vi "ConvertPairSensorReference.vi"(9 "channels":T2[](array[typedef]), 10 "node properties":T1[](array[typedef]), 11 "chan properties in":T1[](array[typedef])) -> (3 "chan properties out":T1[](array[typedef]))   [LabVIEW 2017, in "ServerComm.lvlib"]
uses:
  <vilib>/addons/InsightCM/Devices/Shared/Common/ServerComm/ServerComm.lvlib
  <vilib>/addons/InsightCM/MessageBus/Base/controls/R2_Channel.ctl
  <vilib>/addons/InsightCM/MessageBus/Base/controls/KeyValuePair.ctl
  <vilib>/addons/InsightCM/MessageBus/Base/controls/Metric.ctl
  <vilib>/addons/InsightCM/Utilities/PropertyHelpers/PropertyHelpers.lvlib
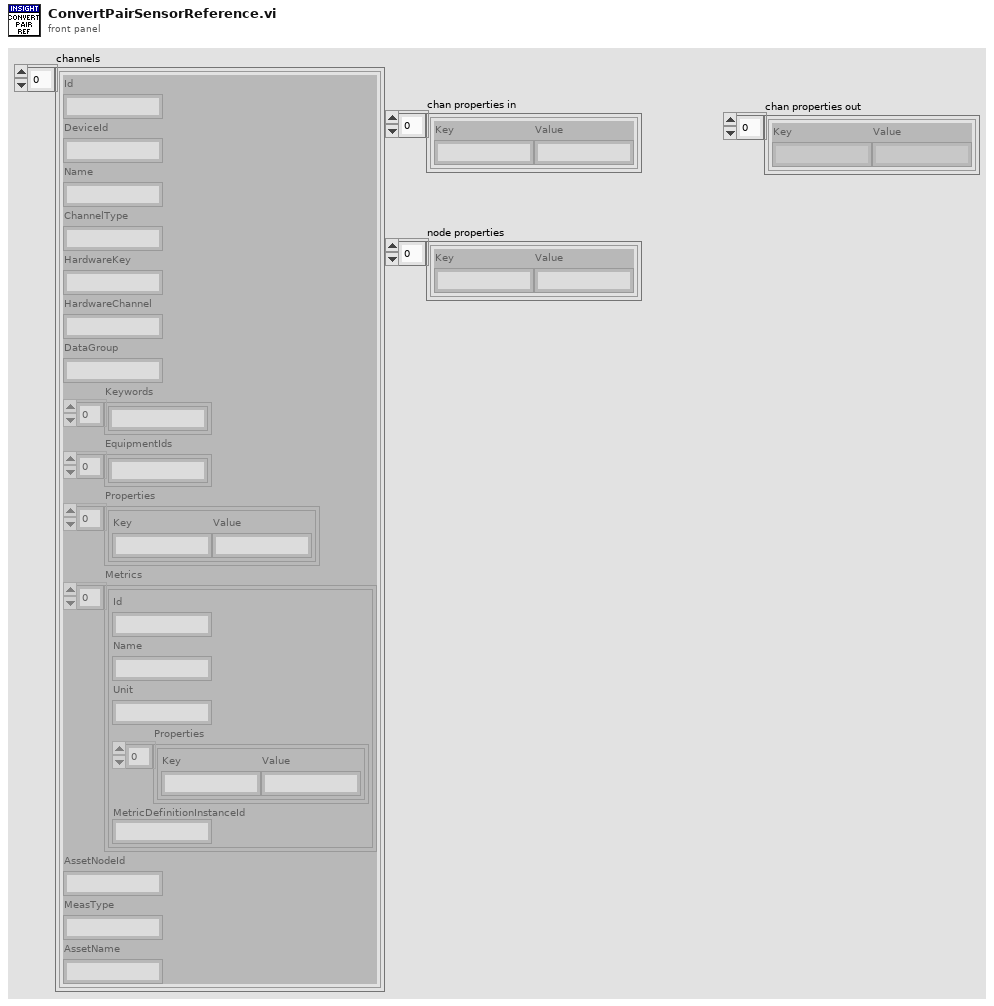
[diagram p1: front panel]
types:
  T1 = typedef "KeyValuePair.ctl" = cluster{"Key":string, "Value":string}
  T2 = typedef "R2_Channel.ctl" = cluster{"Id":string, "DeviceId":string, "Name":string, "ChannelType":string, "HardwareKey":string, "HardwareChannel":string, "DataGroup":string, "Keywords":string[], "EquipmentIds":string[], "Properties":T1[], "Metrics":T3[], "AssetNodeId":string, "MeasType":string, "AssetName":string}
  T3 = typedef "Metric.ctl" = cluster{"Id":string, "Name":string, "Unit":string, "Properties":T1[], "MetricDefinitionInstanceId":string}
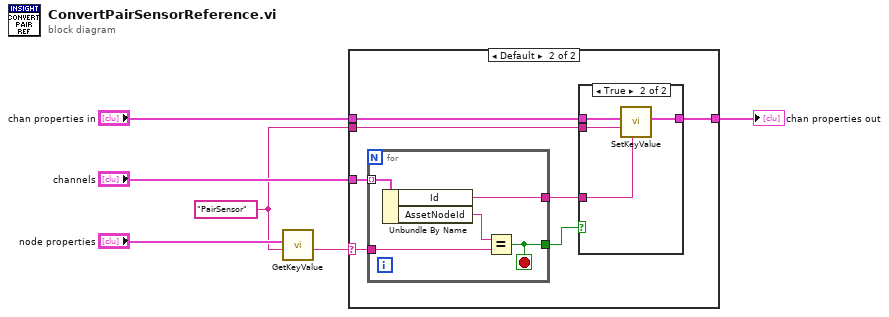
[diagram p0: block diagram]
diagram:
  w2 = "PairSensor" ("key")
  n1 = call <vilib>:"GetKeyValue.vi"("key"=w2, "key value pairs"="node properties") -> ("value"=w4:string)  [unwired: 7 in, 2 out]
  n2 = case shown="Default" w4 {
    selector: w4 -> [_ w13]
    tunnel: "channels" -> [_ w14]
    tunnel: "chan properties in" -> [w7 w11]
    tunnel: w2 -> [_ w10]
    tunnel: [w7 w8] -> w1
    frame "" {
    }
    frame Default {
      n3 = for {
        tunnel: w14 -> [w24] mode=indexing
        tunnel: w13 -> [w22]
        tunnel: [w21] -> w12
        tunnel: [w20] -> w9
        stop <- w21 stop-if-true
        n4 = Unbundle By Name(w24) -> ("Id"=w20:string, "AssetNodeId"=w23:string)
        n5 = Equal?(x=w23, y=w22) -> (x = y?=w21:bool)
      }
      n6 = case shown="True" w12 {
        tunnel: w11 -> [w15 w19]
        tunnel: w10 -> [_ w18]
        tunnel: w9 -> [_ w17]
        tunnel: [w15 w16] -> w8
        frame False {
        }
        frame True {
          n7 = call <vilib>:"SetKeyValue.vi"("value"=w17, "key"=w18, "key value pairs"=w19) -> ("key value pairs out"=w16:T1[])  [unwired: 8 in]
        }
      }
    }
  }
  "chan properties out" <- w1
